vi "Start Logic-Timelapse reminder.vi"(6 "Case name string":string, 8 "error in (no error)":errorcluster, 9 "cancelled":bool) -> (0 "error out":errorcluster)   [LabVIEW 2013]
uses:
  Global Variables/gl_UI Ctrl Refs.vi
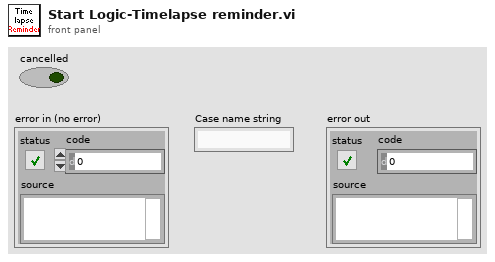
[diagram p1: front panel]
types:
  T1 = typedef "UI ctrl refs cluster.ctl" = cluster{"Top level VI path":path, "Top level VI ref":refnum<vi>, "User menu ref":refnum<k9>, "Sub Panel control":refnum<vi>, "Imaging Param Tab":refnum<vi>, "Occurrence-Start drivers":refnum<k4>, "Occurrence-Speed logging initialised":refnum<k4>, "Occurrence-XYZ stage initialised":refnum<k4>, "Exit button":refnum<vi>, "Status ind":refnum<vi>, "Return to Origin":refnum<vi>, "Speed Logging":refnum<vi>, "Time Lapse":refnum<vi>, "Live Imaging":refnum<vi>, "AOL Z Stack":refnum<vi>, "Motor Z Stack":refnum<vi>, "Funct Acq button":refnum<vi>, "Hard Shutter":refnum<vi>, "Virtual Shutter":refnum<vi>, "Laser Power":refnum<vi>, "AOL Mode":refnum<vi>, "Frame Size":refnum<vi>, "Field of View":refnum<vi>, "Dwell Time":refnum<vi>, "Zoom":refnum<vi>, "AOL Z":refnum<vi>, "Objective":refnum<vi>, "Axis":refnum<vi>, "Paths & Names":refnum<vi>, "Experiment folder path (ind.)":refnum<vi>, "Last State (Ind.)":refnum<vi>, "Laser wavelength ind (nm)":refnum<vi>, "Averages":refnum<vi>, "Angle (degrees)":refnum<vi>, "X centre":refnum<vi>, "Y centre":refnum<vi>, "Plane Mode":refnum<vi>, "# Planes":refnum<vi>, "Z Start":refnum<vi>, "Z Stop":refnum<vi>, "Z Step":refnum<vi>, "PMT 1":refnum<vi>, "PMT 2":refnum<vi>, "Stage XYZ Position":refnum<vi>, "Pockels@Z Start":refnum<vi>, "Pockels@Z Stop":refnum<vi>, "Obtain Z Start":refnum<vi>, "Obtain Z Stop":refnum<vi>, "Live stim.trig.period":refnum<vi>, "Live stim.trig.enable":refnum<vi>, "Funct. Acq. Pockels Modulation":refnum<vi>, "Enable Video Recording":refnum<vi>, "Video Record-Live Imaging":refnum<vi>, "Video Record-Funct acq":refnum<vi>, "AOL Z-stack Chirps Ready (ind)":refnum<vi>, "Center freq ind (nm)":refnum<vi>, "Logging queue (ind)":refnum<vi>, "Back aperture power (ind.)":refnum<vi>, "Power after objective (ind.)":refnum<vi>, "Switch user":refnum<vi>}
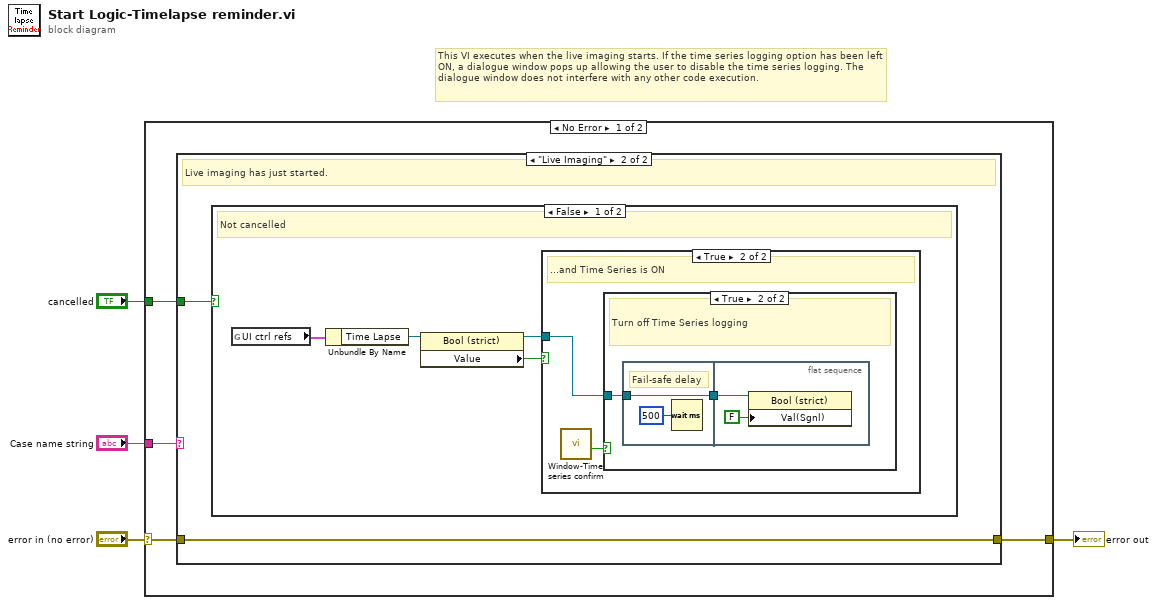
[diagram p0: block diagram]
diagram:
  # "This VI executes when the live imaging starts. If the time series logging option has been left ON, a dialogue window pops up allowing the user to disable the time series logging. The dialogue window does not interfere with any other code execution."
  n1 = case shown="No Error" "error in (no error)" {
    selector: "error in (no error)" -> [w5 w24]
    tunnel: "cancelled" -> [w8 _]
    tunnel: "Case name string" -> [w7 _]
    tunnel: [w6 w24] -> w2
    frame No Error {
      n2 = case shown="\"Live Imaging\"" w7 {
        tunnel: [w9 w11] -> w6
        tunnel: w5 -> [w9 w11]
        tunnel: w8 -> [_ w10]
        frame Default {
        }
        frame "Live Imaging" {
          # "Live imaging has just started."
          n3 = case shown="False" w10 {
            frame False {
              # "Not cancelled"
              n4 = global read "gl_UI Ctrl Refs.vi" "UI ctrl refs"() -> (w13:T1)
              n5 = Unbundle By Name(w13) -> ("Time Lapse"=w15:refnum<vi>)
              n6 = property class="Bool (strict)"(reference=w15) -> (reference out=w12:refnum<vi>, "Value"=w14:bool)  [unwired: 1 in, 1 out]
              n7 = case shown="True" w14 {
                tunnel: w12 -> [_ w16]
                frame False {
                  # "...and Time Series is OFF"
                }
                frame True {
                  # "...and Time Series is ON"
                  n8 = call "Window-Time series confirm.vi"() -> ("Cancelled (Left button pressed)"=w17:bool)  [unwired: 9 in, 2 out]
                  n9 = case shown="True" w17 {
                    tunnel: w16 -> [_ w19]
                    frame False {
                    }
                    frame True {
                      # "Turn off Time Series logging"
                      n10 = flat-sequence {
                        tunnel: w19 -> [w21]
                        tunnel: [w21] -> w18
                        tunnel: w18 -> [w23]
                        frame #0 {
                          # "Fail-safe delay"
                          n11 = Wait (ms)(milliseconds to wait=u32 500) -> ()  [unwired: 1 out]
                        }
                        frame #1 {
                          n12 = property class="Bool (strict)"(reference=w23, "Val(Sgnl)"=FALSE ("Value (Signaling)")) -> ()  [unwired: 1 in, 2 out]
                        }
                      }
                    }
                  }
                }
              }
            }
            frame True {
              # "Cancelled"
            }
          }
        }
      }
    }
    frame Error {
    }
  }
  "error out" <- w2
